vi "Check_Trigger.vi"(0 "Timeout":dbl, 1 "Mode":enum8{"Normal", "Auto", "Auto Level", ""}(ring), 5 "instrument handle In":refnum<k15>, 7 "channelList":string="0", 9 "wfm info in":T1(array[cluster]), 11 "wfm In":i8[][](array[numeric]), 12 "error IN":errorcluster, 14 "Data could not be fetched":bool) -> (3 "Immediate trigged":bool, 4 "wfm info":T1(array[cluster]), 6 "wfm":i8[][](array[numeric]), 8 "error out":errorcluster, 10 "instrument handle out":refnum<k15>, 15 "Time out (False when no trigger is found)":bool)   [LabVIEW 2011]
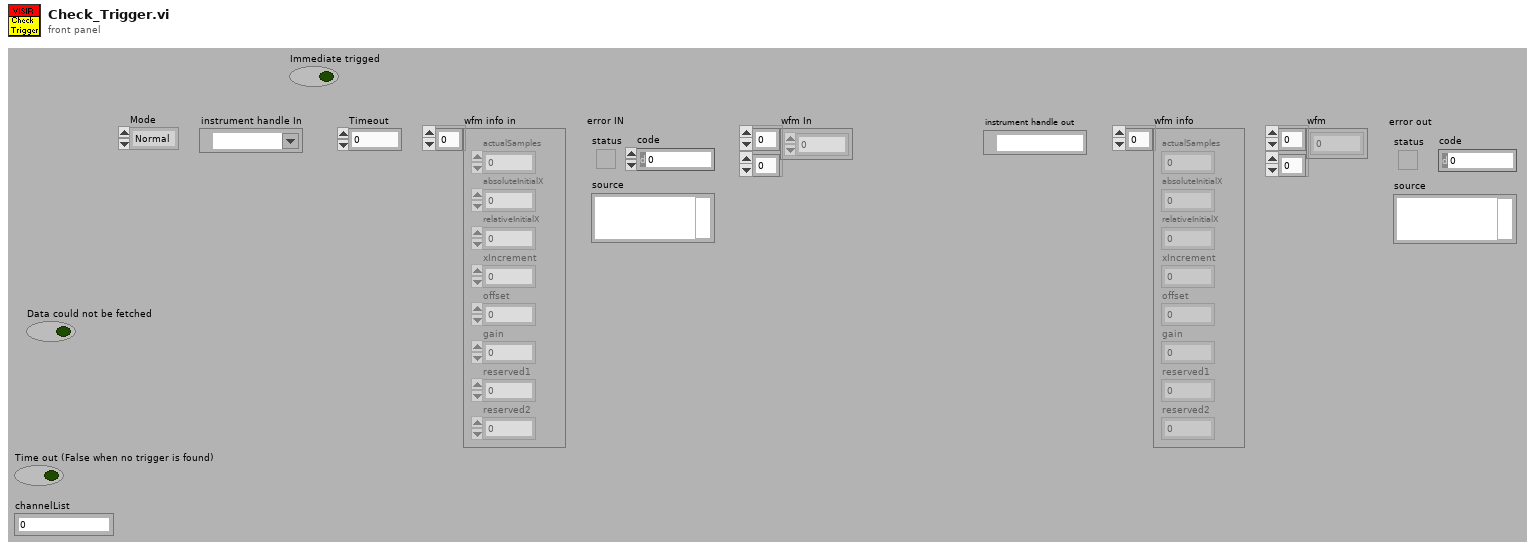
[diagram p1: front panel]
types:
  T1 = cluster{"actualSamples":i32, "absoluteInitialX":dbl, "relativeInitialX":dbl, "xIncrement":dbl, "offset":dbl, "gain":dbl, "reserved1":dbl, "reserved2":dbl}[]
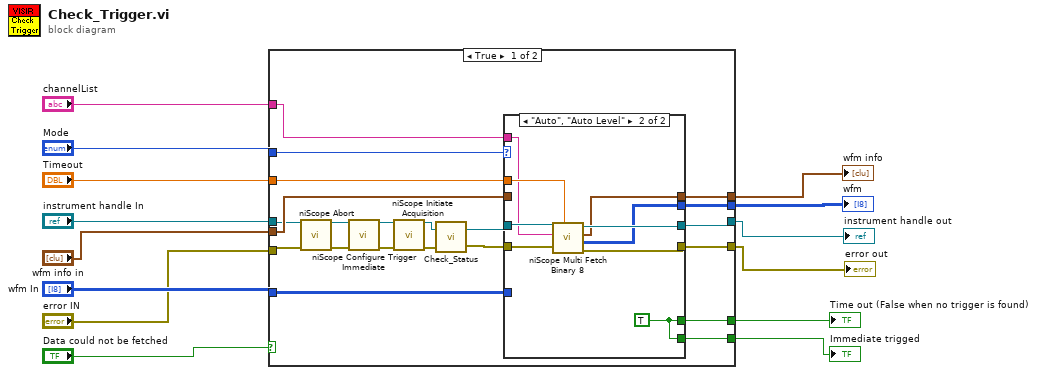
[diagram p0: block diagram]
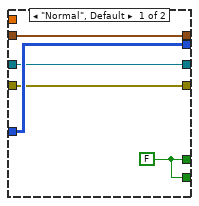
[diagram p2: hidden frame]
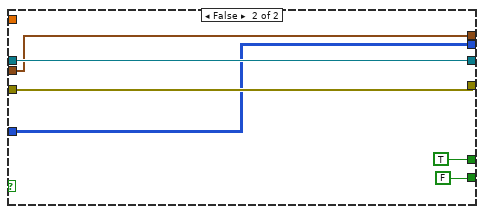
[diagram p3: hidden frame]
diagram:
  n1 = case shown="True" "Data could not be fetched" {
    tunnel: [w34 w55] -> w12
    tunnel: "instrument handle In" -> [w23 w55]
    tunnel: [w33 w54] -> w11
    tunnel: "error IN" -> [w22 w54]
    tunnel: [w30 w53] -> w13
    tunnel: "wfm info in" -> [w29 w53]
    tunnel: [w32 w52] -> w10
    tunnel: "wfm In" -> [w31 w52]
    tunnel: "Mode" -> [w35 _]
    tunnel: "Timeout" -> [w28 _]
    tunnel: [w21 TRUE] -> w4
    tunnel: "channelList" -> [w16 _]
    tunnel: [w15 FALSE] -> w1
    frame True {
      n2 = call <instrlib>:"niScope Abort.vi"("instrument handle"=w23, "error in"=w22) -> ("instrument handle out"=w27:refnum<k15>, "error out"=w24:errorcluster)  [unwired: 12 in]
      n3 = call <instrlib>:"niScope Configure Trigger Immediate.vi"("instrument handle"=w27, "error in"=w24) -> ("instrument handle out"=w26:refnum<k15>, "error out"=w25:errorcluster)  [unwired: 12 in]
      n4 = call <instrlib>:"niScope Initiate Acquisition.vi"("instrument handle"=w26, "error in"=w25) -> ("instrument handle out"=w20:refnum<k15>, "error out"=w17:errorcluster)  [unwired: 12 in]
      n5 = call "Check_Status.vi"("error in"=w17, "instrument handle in"=w20) -> ("error out"=w18:errorcluster, "instrument handle out"=w19:refnum<k15>)
      n6 = case shown="\"Auto\", \"Auto Level\"" w35 {
        tunnel: [w38 w48] -> w34
        tunnel: [w37 w45] -> w33
        tunnel: [w40 w46] -> w32
        tunnel: w31 -> [w40 _]
        tunnel: [w39 w47] -> w30
        tunnel: w29 -> [w39 _]
        tunnel: w28 -> [_ w49]
        tunnel: w19 -> [w38 w44]
        tunnel: w18 -> [w37 w42]
        tunnel: [w36 w41] -> w21
        tunnel: w16 -> [_ w43]
        tunnel: [w36 w41] -> w15
        frame "Normal", Default {
          w36 = FALSE
        }
        frame "Auto", "Auto Level" {
          w41 = TRUE
          n7 = call <instrlib>:"niScope Multi Fetch Binary 8.vi"("timeout"=w49, "error in"=w42, "channels"=w43, "instrument handle"=w44) -> ("error out"=w45:errorcluster, "wfm"=w46:i8[][], "wfm info"=w47:T1, "instrument handle out"=w48:refnum<k15>)  [unwired: 4 in]
        }
      }
    }
    frame False {
    }
  }
  "wfm info" <- w13
  "instrument handle out" <- w12
  "error out" <- w11
  "wfm" <- w10
  "Time out (False when no trigger is found)" <- w4
  "Immediate trigged" <- w1
